vi "main.vi"(8 "error in (no error)":errorcluster, 11 "DinnerSimulator in":refnum<class "DinnerSimulator.lvclass">) -> (0 "error out":errorcluster, 3 "DinnerSimulator out":refnum<class "DinnerSimulator.lvclass">)   [LabVIEW 2011, in "DinnerSimulator.lvclass"]
uses:
  DinnerSimulator.lvclass
  Kitchen/Kitchen.lvclass
  CookBehaviors/Pop/Pop.lvclass
  Appliances/PopcornPopper/PopcornPopper.lvclass
  Appliances/Oven/Oven.lvclass
  CookBehaviors/Bake/Bake.lvclass
  CookBehaviors/Simmer/Simmer.lvclass
  Appliances/Stove/Stove.lvclass
  Appliance/Appliance.lvclass
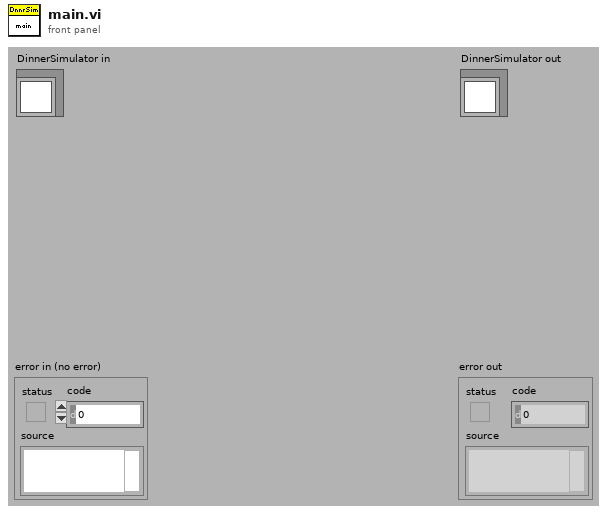
[diagram p1: front panel]
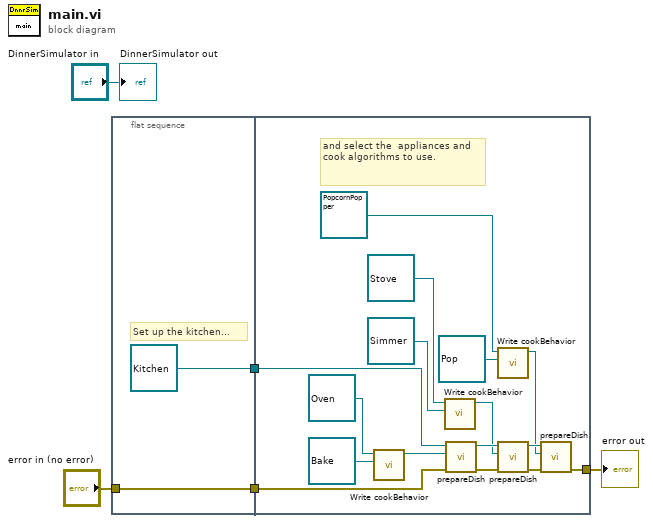
[diagram p0: block diagram]
diagram:
  n1 = flat-sequence {
    tunnel: [w7] -> w4
    tunnel: "error in (no error)" -> [w7]
    tunnel: [refnum<class "Kitchen.lvclass"> refnum ("Kitchen.lvclass")] -> w1
    tunnel: w4 -> [w21]
    tunnel: [w18] -> w2
    tunnel: w1 -> [w8]
    frame #0 {
      # "Set up the kitchen..."
    }
    frame #1 {
      # "and select the  appliances and cook algorithms to use."
      n2 = call "Write cookBehavior.vi"("cookBehavior"=refnum<class "Bake.lvclass"> refnum ("CookBehaviors.lvlib:Bake.lvclass"), "Appliance in"=refnum<class "Oven.lvclass"> refnum ("Appliances.lvlib:Oven.lvclass")) -> ("Appliance out"=w9:refnum<class "Oven.lvclass">)  [unwired: 8 in, 1 out]
      n3 = call "Write cookBehavior.vi"("cookBehavior"=refnum<class "Simmer.lvclass"> refnum ("CookBehaviors.lvlib:Simmer.lvclass"), "Appliance in"=refnum<class "Stove.lvclass"> refnum ("Appliances.lvlib:Stove.lvclass")) -> ("Appliance out"=w10:refnum<class "Stove.lvclass">)  [unwired: 8 in, 1 out]
      n4 = call "prepareDish.vi"("error in (no error)"=w21, "appliance"=w9, "Kitchen in"=w8) -> ("error out"=w20:errorcluster, "Kitchen out"=w22:refnum<class "Kitchen.lvclass">)  [unwired: 7 in]
      n5 = call "Write cookBehavior.vi"("cookBehavior"=refnum<class "Pop.lvclass"> refnum ("CookBehaviors.lvlib:Pop.lvclass"), "Appliance in"=refnum<class "PopcornPopper.lvclass"> refnum ("Appliances.lvlib:PopcornPopper.lvclass")) -> ("Appliance out"=w11:refnum<class "PopcornPopper.lvclass">)  [unwired: 8 in, 1 out]
      n6 = call "prepareDish.vi"("error in (no error)"=w20, "appliance"=w10, "Kitchen in"=w22) -> ("error out"=w19:errorcluster, "Kitchen out"=w23:refnum<class "Kitchen.lvclass">)  [unwired: 7 in]
      n7 = call "prepareDish.vi"("error in (no error)"=w19, "appliance"=w11, "Kitchen in"=w23) -> ("error out"=w18:errorcluster)  [unwired: 7 in, 1 out]
    }
  }
  "error out" <- w2
  "DinnerSimulator out" <- "DinnerSimulator in"
